vi "Text Operations on Labview.vi"() -> ()   [LabVIEW 2024]
panel:
  in  "Input Text":string
  in  "access (0:read/write)":enum16{"read/write", "read-only", "write-only"}(ring)
  in  "file path (use dialog)":path
  in  "stop":bool
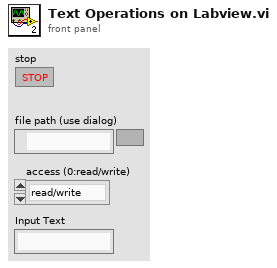
[diagram p1: front panel]
types:
  T1 = enum16{"open", "replace", "create", "open or create", "replace or create", "replace or create with confirmation"}
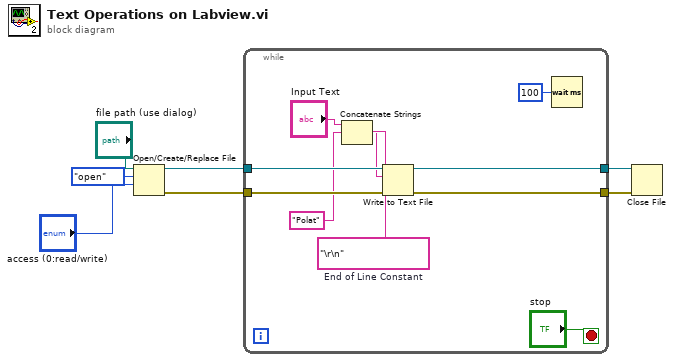
[diagram p0: block diagram]
diagram:
  n1 = Open/Create/Replace File(file path (use dialog)="file path (use dialog)", operation (0:open)=T1."open", access (0:read/write)="access (0:read/write)") -> (refnum out=w2:refnum<file>, error out=w4:errorcluster)  [unwired: 3 in, 1 out]
  n2 = while {
    tunnel: w4 -> [w16]
    tunnel: [w15] -> w3
    tunnel: w2 -> [w14]
    tunnel: [w13] -> w1
    stop <- "stop" stop-if-true
    w9 = "\r\n"  # End of Line Constant
    n3 = Concatenate Strings "Concatenate Strings"("Input Text", "Polat", w9) -> (w8:string)
    n4 = Write to Text File(file (use dialog)=w14, text=w8, error in=w16) -> (refnum out=w13:refnum<file>, error out=w15:errorcluster)  [unwired: 1 in, 1 out]
    n5 = Wait (ms)(milliseconds to wait=u32 100) -> ()  [unwired: 1 out]
  }
  n6 = Close File(refnum=w1, error in=w3) -> ()  [unwired: 2 out]
